vi "Do.vi"(8 "error in":errorcluster, 10 "Actor in":refnum<class "Actor.lvclass">, 11 "Change PID Controls MSG":refnum<class "Change PID Controls MSG.lvclass">) -> (0 "error out":errorcluster, 2 "Actor out":refnum<class "Actor.lvclass">)   [LabVIEW 2014, in "Change PID Controls MSG.lvclass"]
doc: "(<B>Filename</B>: Actor Framework.lvlib:Message.lvclass:Do.vi)\n\nDefines what a message does when it is received by an actor. Generally, a message instructs an actor to invoke one of its methods. By default, this method does nothing. A child class must override it to define behavior. Create a child class by using the Actor Framework Message Maker dialog box."
uses:
  Change PID Controls MSG.lvclass
  <vilib>/ActorFramework/Actor/Actor.lvclass
  reusable/DAQ Device/Device/Device.lvclass
  TE Cooler.lvclass
  reusable/DAQ Device/Device/Device.lvclass/Device.ctl
  SuperActor/SuperActor.lvclass/SuperActor.ctl
  Change PID Controls MSG.lvclass/Change PID Controls MSG.ctl
  reusable/DAQ Device/Device/Read Configurable Device.vi
  SuperActor/Read CVT Session.vi
  SuperActor/Read Log Session.vi
  SuperActor/Read ID.vi
  Configurable Device/Configurable Device.lvclass
  <userlib>/_Session Fwk/Session - Root.lvclass
  reusable/Session APIs/Session Log/System Log.lvclass
  reusable/Session APIs/CVT/CVT.lvclass
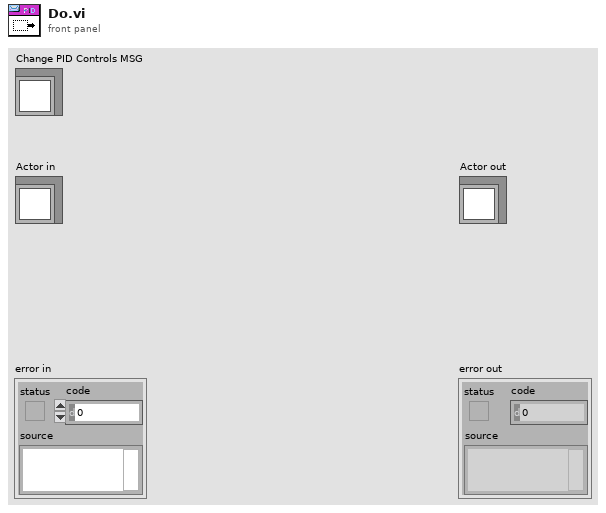
[diagram p1: front panel]
types:
  T1 = typedef "Session - Root.lvclass/Session Handle.ctl" = refnum<data-value>
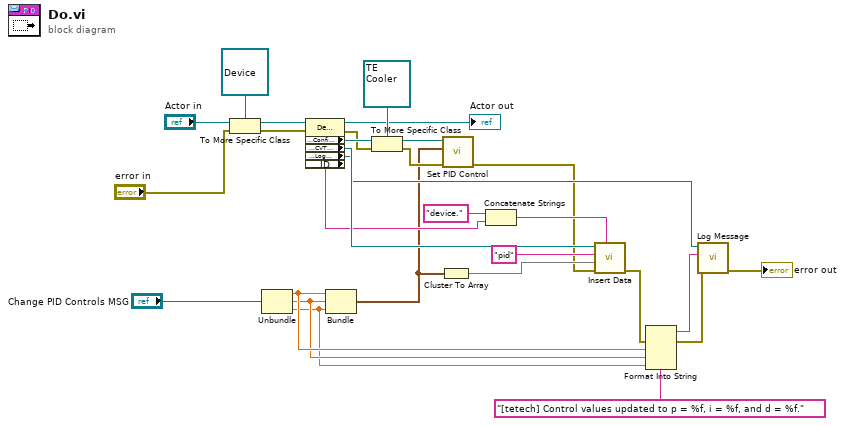
[diagram p0: block diagram]
diagram:
  n1 = To More Specific Class(target class=refnum<class "Device.lvclass"> refnum ("DAQ Device.lvlib:Device"), reference="Actor in", error in="error in") -> (specific class reference=w26:refnum<class "Device.lvclass">, error out=w25:errorcluster)
  n2 = Unbundle("Change PID Controls MSG") -> (w7:dbl, w6:dbl, w5:dbl)
  n3 = property class="Device"(reference=w26, error in=w25) -> (reference out=→"Actor out":refnum<class "Device.lvclass">, error out=w19:errorcluster, "Accessors:Configurable Device"=w24:refnum<class "Configurable Device.lvclass">, "Accessors:CVT Session"=w18:T1, "Accessors:Log Session"=w17:T1, "Accessors:ID"=w15:string)
  n4 = Bundle("P"=w7, "I"=w6, "D"=w5) -> (w12:cluster{"P":dbl, "I":dbl, "D":dbl})  [unwired: 1 in]
  n5 = To More Specific Class(target class=refnum<class "TE Cooler.lvclass"> refnum ("TE Cooler.lvlib:TE Tech"), reference=w24, error in=w19) -> (specific class reference=w22:refnum<class "TE Cooler.lvclass">, error out=w20:errorcluster)
  n6 = Cluster To Array(cluster=w12) -> (array=w11:dbl[])
  n7 = call "Set PID Control.vi"("error in"=w20, "Ctl Vals"=w12, "TE Cooler in"=w22) -> ("error out"=w10:errorcluster)  [unwired: 7 in, 1 out]
  n8 = Concatenate Strings("device." ("string"), w15) -> (w14:string)
  n9 = call "Insert Data.vi"("Group"=w14, "error in"=w10, "Data"=w11, "tag"="pid", "CVT Session In"=w18) -> ("error out"=w2:errorcluster)  [unwired: 5 in, 1 out]
  n10 = Format Into String(format string="[tetech] Control values updated to p = %f, i = %f, and d = %f.", error in=w2, w7, w6, w5) -> (resulting string=w4:string, error out=w1:errorcluster)  [unwired: 1 in]
  n11 = call "Log Message.vi"("error in"=w1, "MSG In"=w4, "session in"=w17) -> ("error out"=→"error out":errorcluster)  [unwired: 7 in, 1 out]
